vi "Get_LV_values_from_PS.vi"(8 "error in (no error)":errorcluster, 11 "Response":string) -> (0 "error out":errorcluster, 1 "Content":string, 2 "Headers":cluster{"Name":string, "Value":string}[](array[cluster]), 3 "Status Description":string, 4 "Errors":string, 5 "Status Code":i32)   [LabVIEW 2016, in "Response.lvclass"]
uses:
  Response.lvclass
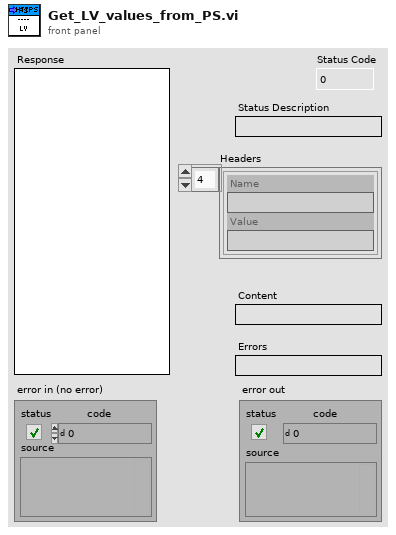
[diagram p1: front panel]
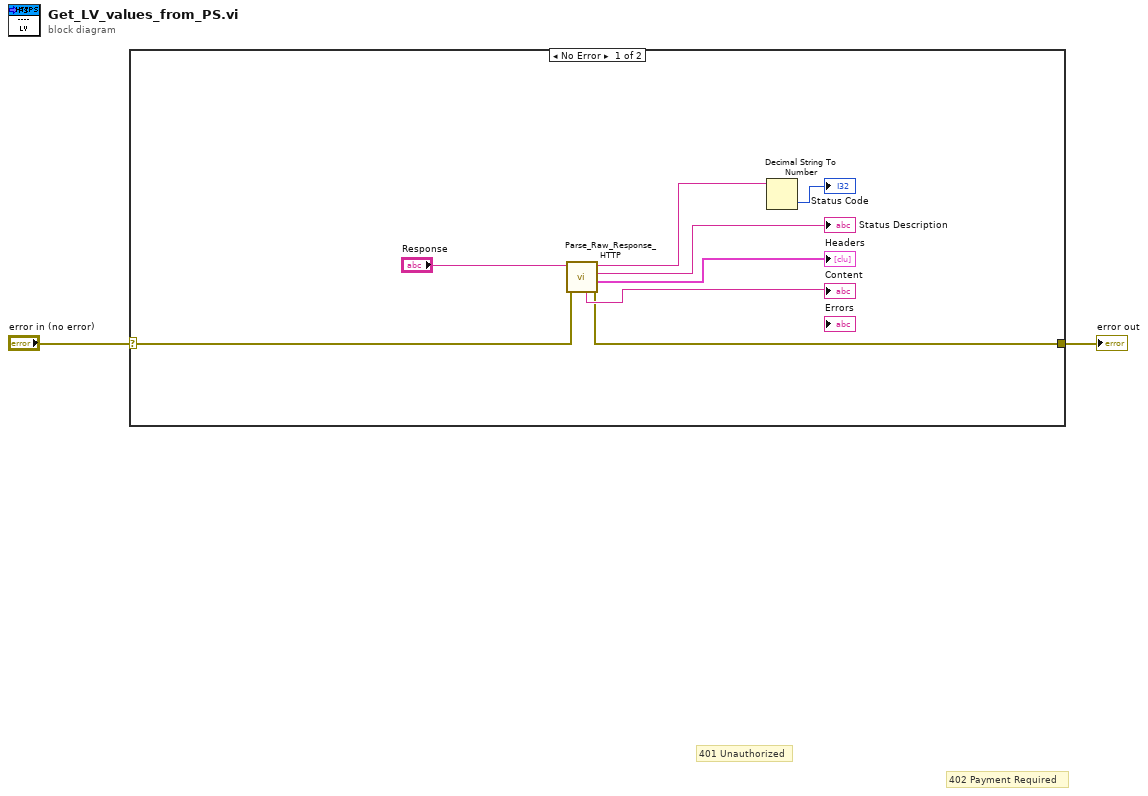
[diagram p0: block diagram]
diagram:
  # "402 Payment Required"
  # "401 Unauthorized"
  n1 = case shown="No Error" "error in (no error)" {
    selector: "error in (no error)" -> [w4 w11]
    tunnel: [w3 w11] -> w2
    frame No Error {
      n2 = call "Parse_Raw_Response_HTTP.vi"("error in (no error)"=w4, "HTTP Response"="Response") -> ("error out"=w3:errorcluster, "Headers"=→"Headers":cluster{"Name":string, "Value":string}[], "Status Description"=→"Status Description":string, "Status Code"=w7:string, "Body"=→"Content":string)  [unwired: 5 in]
      n3 = Decimal String To Number(string=w7) -> (number=→"Status Code":i32)  [unwired: 2 in, 1 out]
    }
    frame Error {
    }
  }
  "error out" <- w2
